vi "Read VI Plain Name.vi"(8 "error in (no error)":errorcluster, 11 "VI in":refnum<class "VI.lvclass">) -> (0 "error out":errorcluster, 2 "VI Plain Name":string, 3 "VI out":refnum<class "VI.lvclass">)   [LabVIEW 2019, in "Panther Dashboard.lvlib" / "VI.lvclass"]
uses:
  VI.lvclass
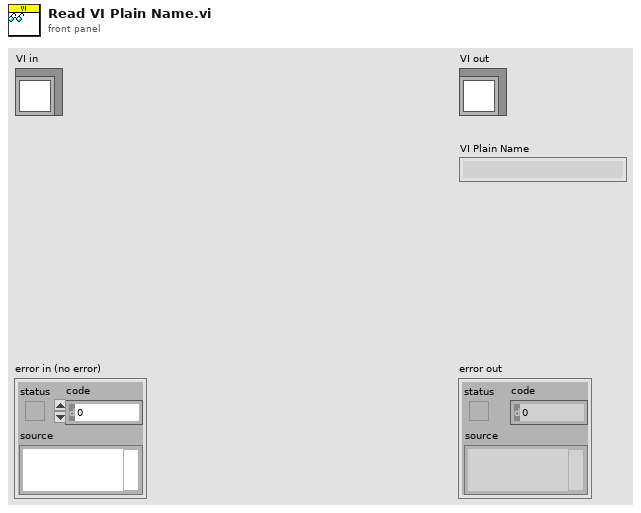
[diagram p1: front panel]
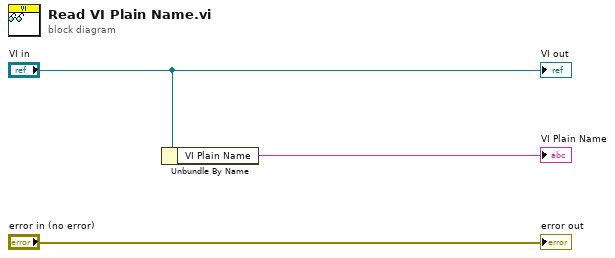
[diagram p0: block diagram]
diagram:
  n1 = Unbundle By Name("VI in") -> ("VI Plain Name"=→"VI Plain Name":string)
  "error out" <- "error in (no error)"
  "VI out" <- "VI in"
